vi "Read Parameters.vi"(8 "error in (no error)":errorcluster, 11 "EL-Go To Height in":refnum<class "EL-Go To Height.lvclass">) -> (0 "error out":errorcluster, 2 "Parameters":T1={"Target Height"=0.0, "Elevator State Loop (ms)"=20, "Up Rate (Percentage)"=0.0, "Down Rate (Percentage)"=0.0}, 3 "EL-Go To Height out":refnum<class "EL-Go To Height.lvclass">)   [LabVIEW 2014, in "Elevator.lvlib" / "EL-Go To Height.lvlib" / "EL-Go To Height.lvclass"]
uses:
  EL-Go To Height.lvclass
  Parameters.ctl
  EL-Go To Height.lvclass/EL-Go To Height.ctl
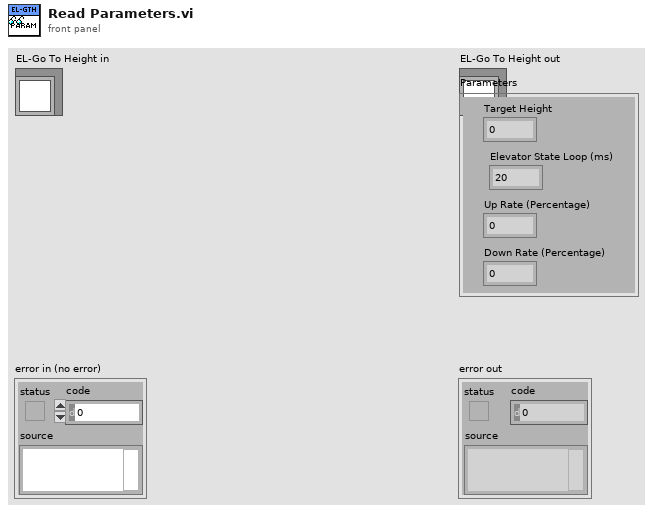
[diagram p1: front panel]
types:
  T1 = typedef "Elevator.lvlib/EL-Go To Height.lvlib/EL-Go To Height.lvclass/Parameters.ctl" = cluster{"Target Height":dbl, "Elevator State Loop (ms)":u32, "Up Rate (Percentage)":dbl, "Down Rate (Percentage)":dbl}
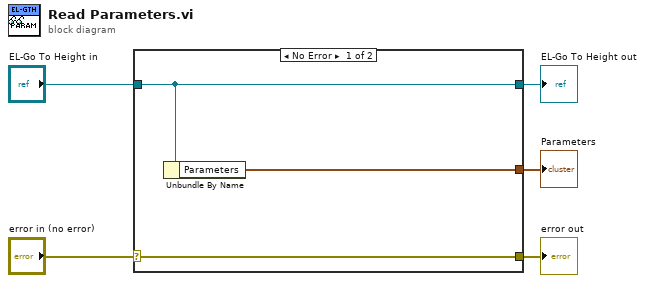
[diagram p0: block diagram]
diagram:
  n1 = case shown="No Error" "error in (no error)" {
    selector: "error in (no error)" -> [w8 w9]
    tunnel: [w8 w9] -> w4
    tunnel: [w7 w10] -> w2
    tunnel: "EL-Go To Height in" -> [w7 w10]
    tunnel: [w6 _] -> w1
    frame No Error {
      n2 = Unbundle By Name(w7) -> ("Parameters"=w6:T1)
    }
    frame Error {
    }
  }
  "error out" <- w4
  "EL-Go To Height out" <- w2
  "Parameters" <- w1
